vi "Read Frequency.vi"(8 "error in (no error)":errorcluster, 11 "build_waveform in":refnum<class "build_waveform.lvclass">) -> (0 "error out":errorcluster, 2 "Frequency":i32=220000000, 3 "build_waveform out":refnum<class "build_waveform.lvclass">)   [LabVIEW 2015, in "build_waveform.lvclass"]
uses:
  build_waveform.lvclass
  build_waveform.lvclass/build_waveform.ctl
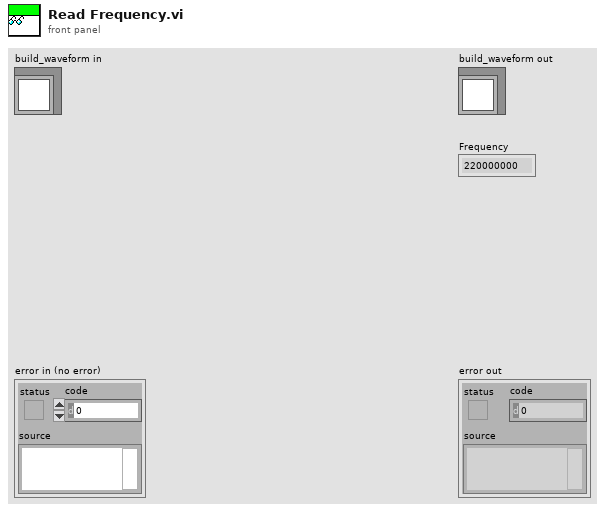
[diagram p1: front panel]
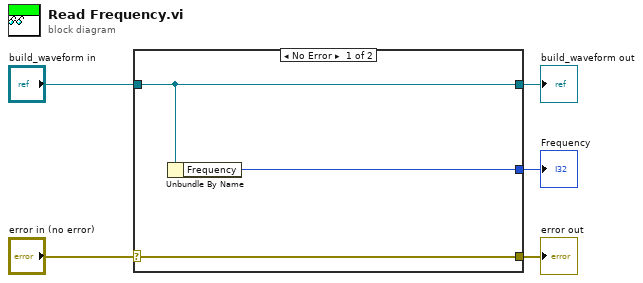
[diagram p0: block diagram]
diagram:
  n1 = case shown="No Error" "error in (no error)" {
    selector: "error in (no error)" -> [w8 w9]
    tunnel: [w8 w9] -> w4
    tunnel: [w7 w10] -> w2
    tunnel: "build_waveform in" -> [w7 w10]
    tunnel: [w6 _] -> w1
    frame No Error {
      n2 = Unbundle By Name(w7) -> ("Frequency"=w6:i32)
    }
    frame Error {
    }
  }
  "error out" <- w4
  "build_waveform out" <- w2
  "Frequency" <- w1
